vi "Initialize Default Values.vi"(8 "error in (no error)":errorcluster, 9 "Initialized?":bool, 10 "Default Control Values in":variant[](array[variant]), 11 "VI in":refnum<vi>) -> (0 "error out":errorcluster, 3 "Default Control Values out":variant[](array[variant]))   [LabVIEW 2013]
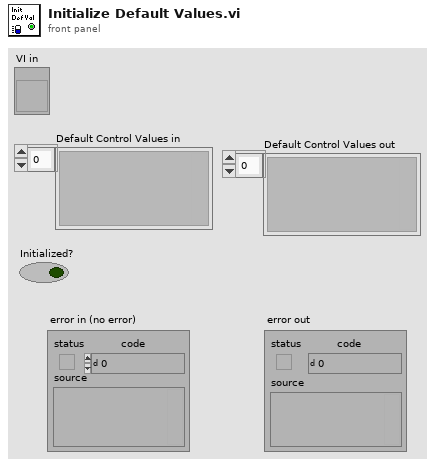
[diagram p1: front panel]
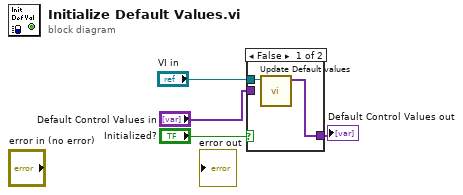
[diagram p0: block diagram]
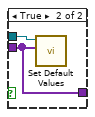
[diagram p2: hidden frame]
diagram:
  n1 = case shown="False" "Initialized?" {
    tunnel: "VI in" -> [w6 w8]
    tunnel: "Default Control Values in" -> [_ w7]
    tunnel: [w5 w7] -> w4
    frame False {
      n2 = call "Update Default values.vi"("VI in"=w6) -> ("Default Values out"=w5:variant[])  [unwired: 10 in]
    }
    frame True {
      n3 = call "Set Default Values.vi"("Default Values in"=w7, "VI in"=w8) -> ()  [unwired: 10 in]
    }
  }
  "Default Control Values out" <- w4
